vi "Command_verification.vi"(0 "connection ID":refnum<k5>, 1 "System \nSelection":enum32{"Common", "Frosk", "Griffin", "K2"}(ring), 3 "Mode":string(combo)="DProbe", 5 "VTxIndex_In":i8, 6 "probeNumElevAper":i32=1, 9 "time out":i32=40000, 11 "elevAperIndex":i8, 12 "TxpgWaveformStyle":i8) -> (4 "Get_mea_condition":T1 {"RoiLateralSpan" format="%.2f"; "RoiLateralMin" format="%.2f"}, 8 "ElevAperSwitchDepth":sgl, 10 "Result_RLE":bool, 14 "RLE data":string, 15 "Control_elevAperSwitch":bool)   [LabVIEW 2016]
panel:
  out "Dmode(Hout_Lout_Reg)":string[](array[string])
  out "error out 2":errorcluster
  in  "mea_condition_setting":T1 {"RoiLateralMin" format="%.2f"; "RoiLateralSpan" format="%.2f"; "pulseVoltage" format="%.2f"}
  in  "error out":errorcluster
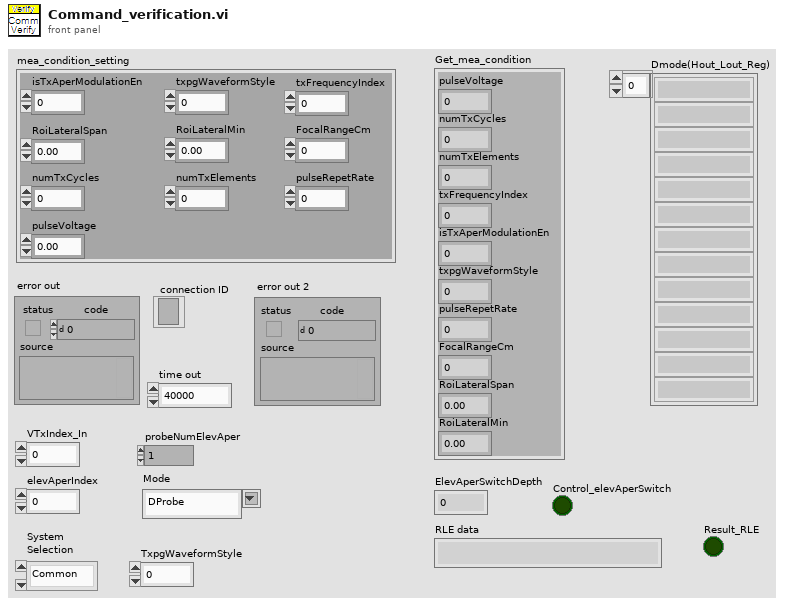
[diagram p1: front panel]
types:
  T1 = cluster{"pulseVoltage":dbl, "numTxCycles":dbl, "numTxElements":i16, "txFrequencyIndex":i32, "isTxAperModulationEn":i16, "txpgWaveformStyle":i16, "pulseRepetRate":dbl, "FocalRangeCm":dbl, "RoiLateralSpan":dbl, "RoiLateralMin":dbl}
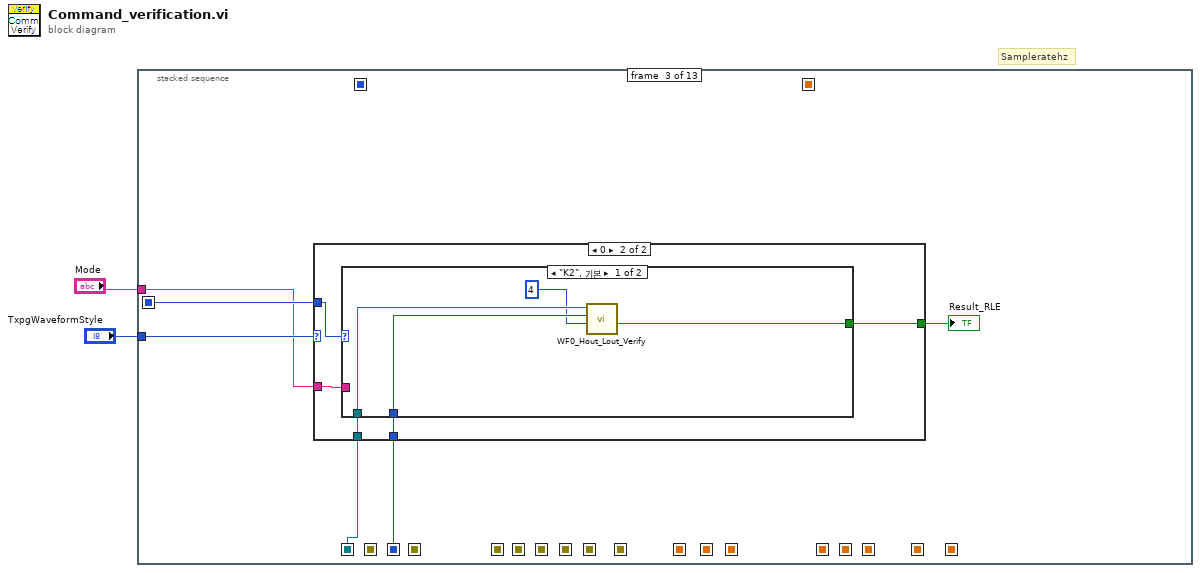
[diagram p0: block diagram]
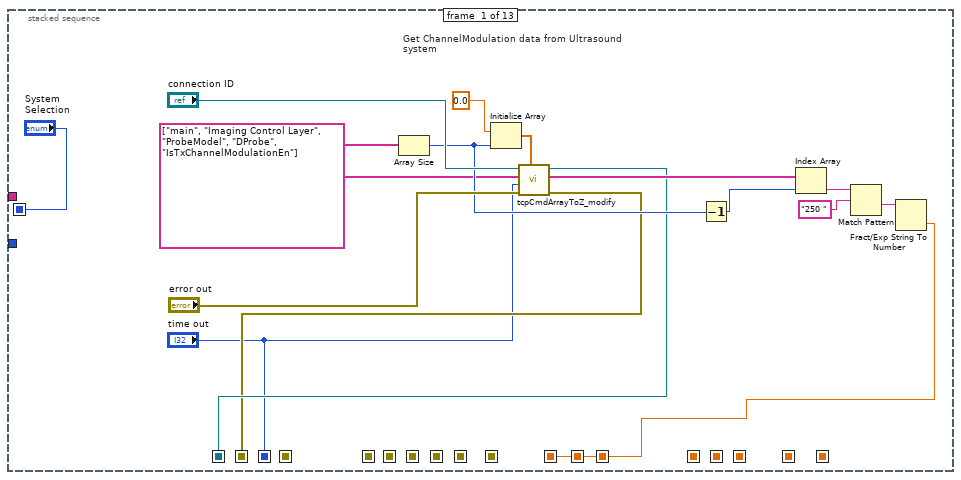
[diagram p2: hidden frame]
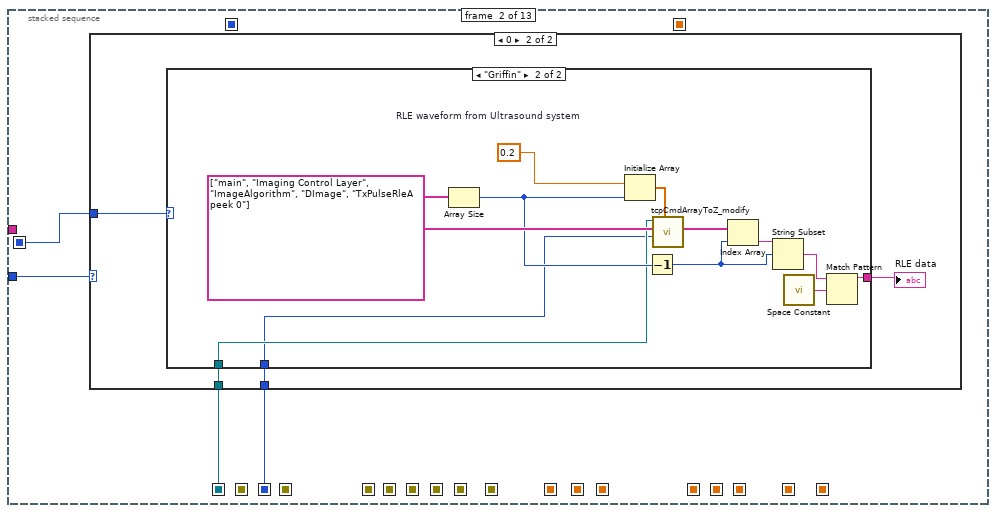
[diagram p3: hidden frame]
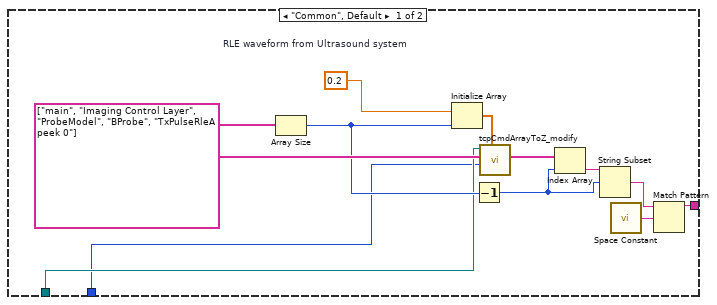
[diagram p5: hidden frame]
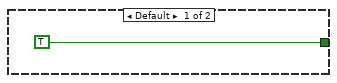
[diagram p6: hidden frame]
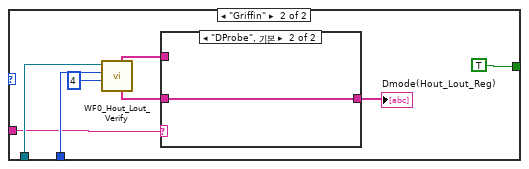
[diagram p7: hidden frame]
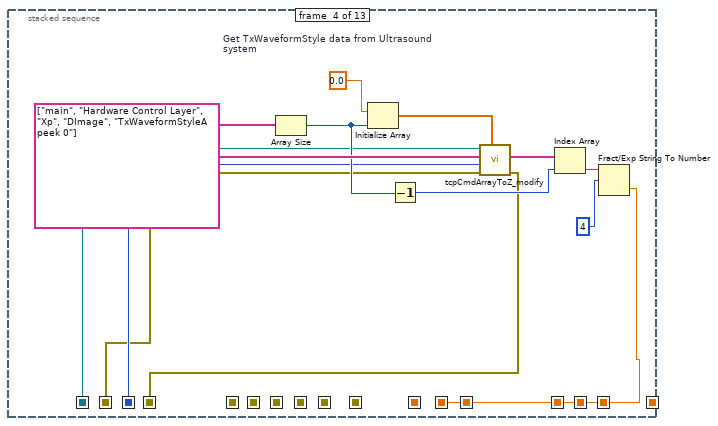
[diagram p9: hidden frame]
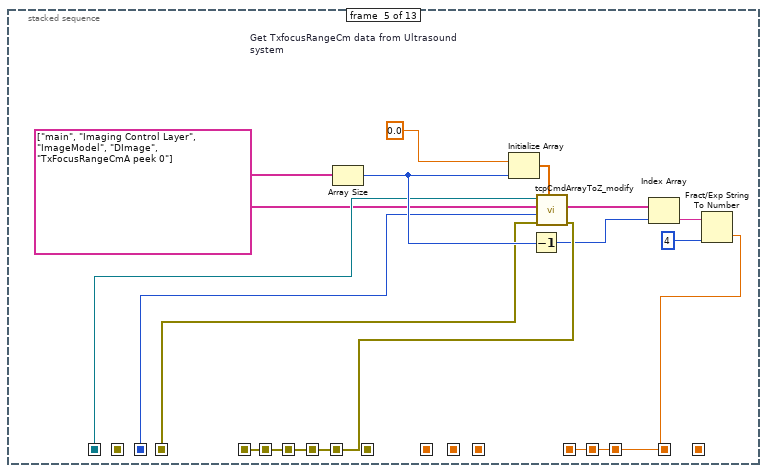
[diagram p10: hidden frame]
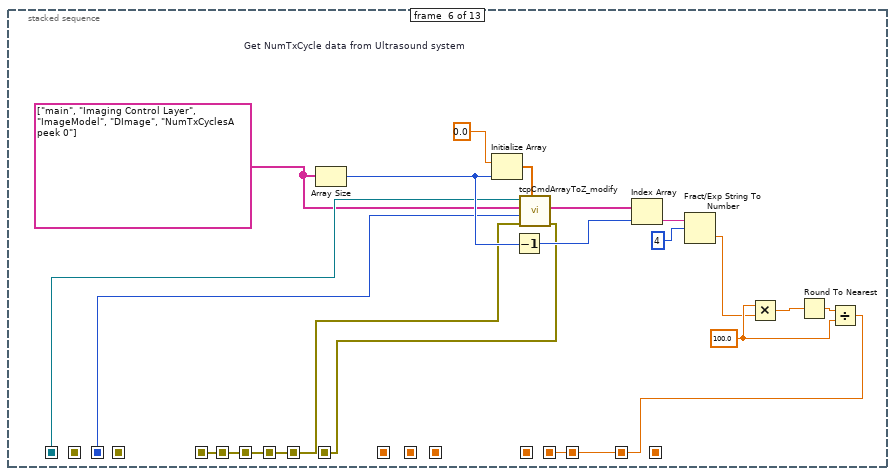
[diagram p11: hidden frame]
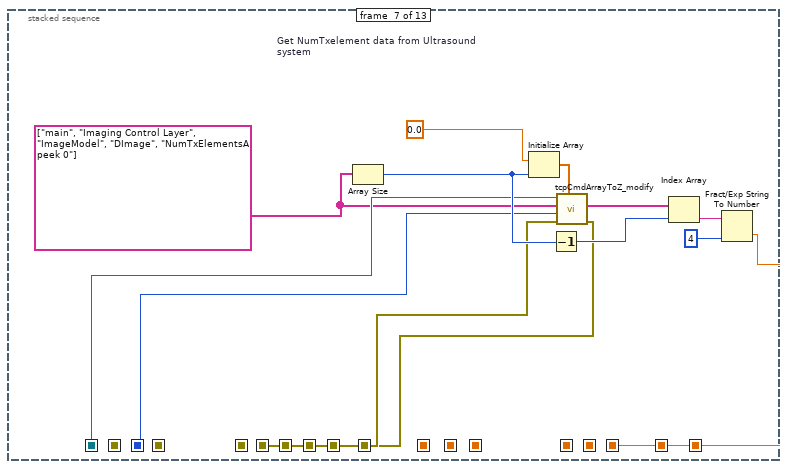
[diagram p12: hidden frame]
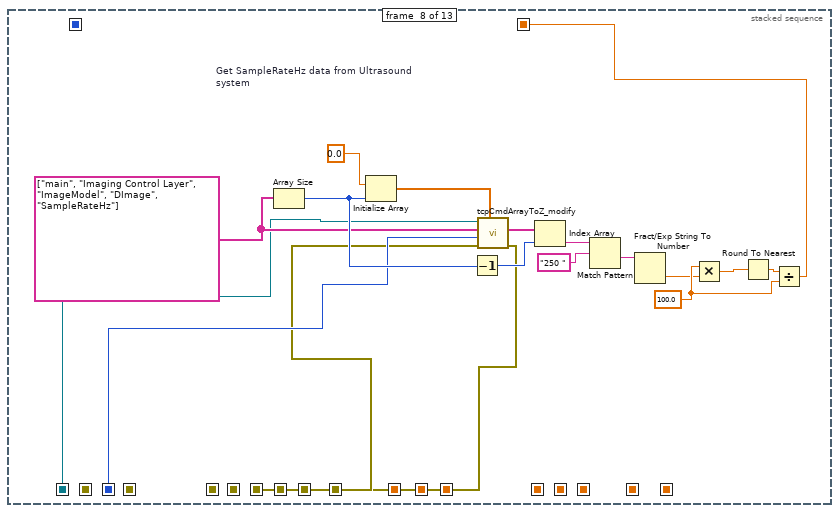
[diagram p13: hidden frame]
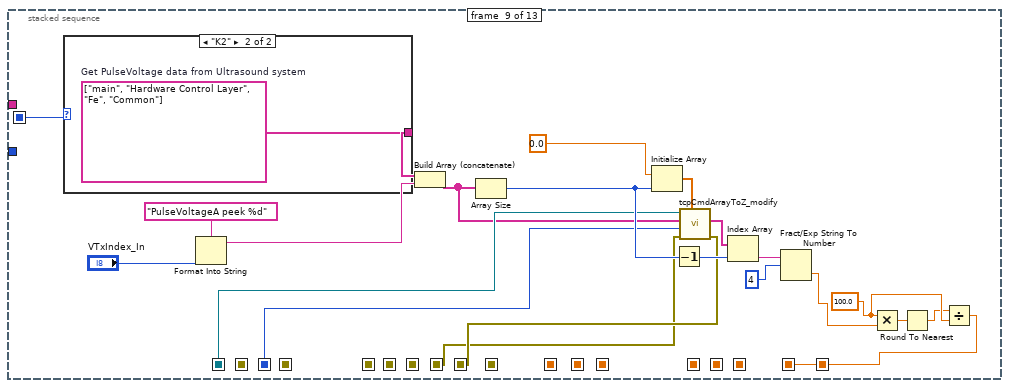
[diagram p14: hidden frame]
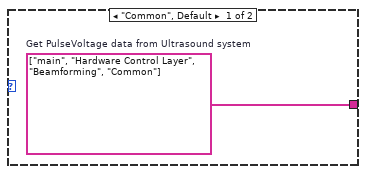
[diagram p15: hidden frame]
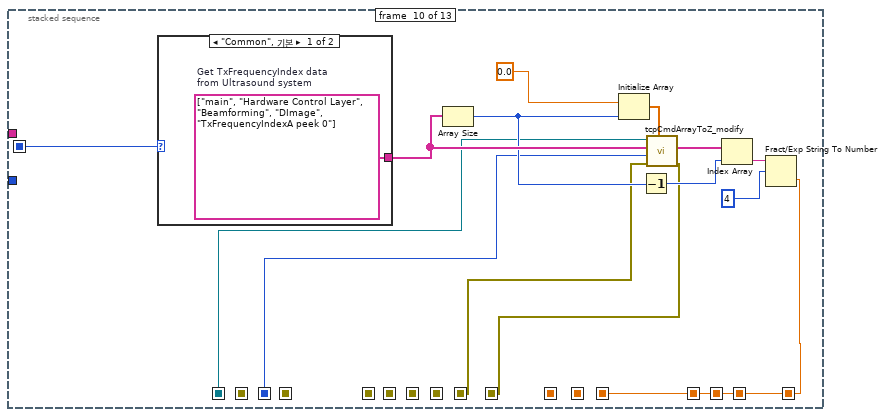
[diagram p16: hidden frame]
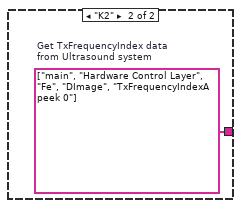
[diagram p17: hidden frame]
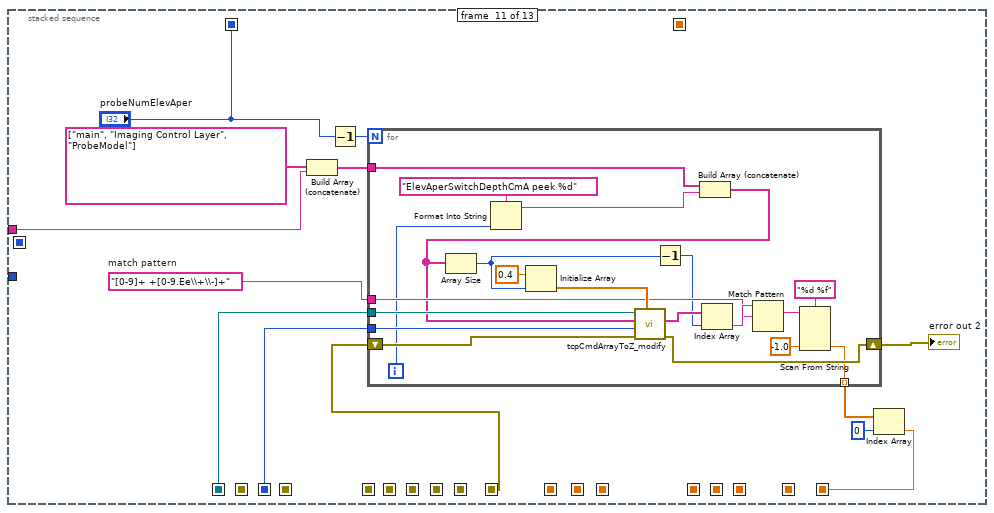
[diagram p18: hidden frame]
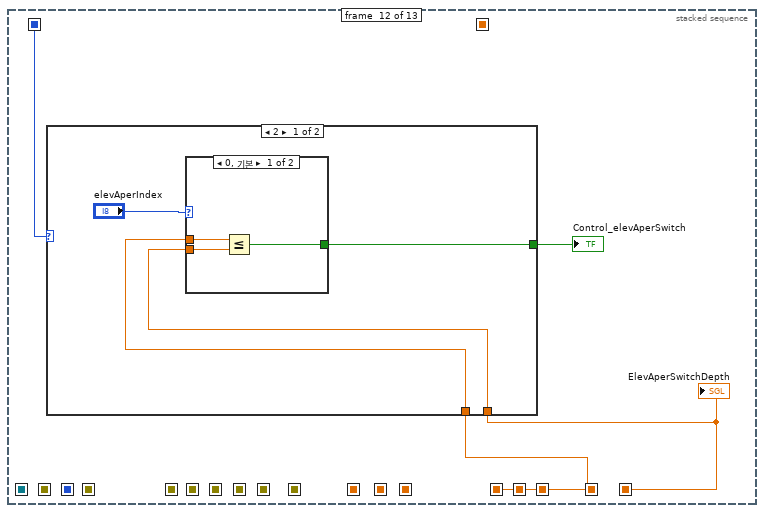
[diagram p19: hidden frame]
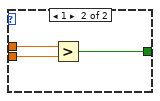
[diagram p20: hidden frame]
diagram:
  # "Sampleratehz"
  n1 = stacked-sequence {
    seq-local: [w11 _ _ _ _ _ _ _ _ _ _ _ _] -> [_ _ _ _ _ _ _ _ _ _ _ _ w247]
    seq-local: [w10 _ _ _ _ _ _ _ _ _ _ _ _] -> [_ w22 w56 w84 w98 w113 w126 w141 w166 w180 w198 _ _]
    seq-local: [w9 _ _ _ _ _ _ _ _ _ _ _ _] -> [_ _ _ w82 _ _ _ _ _ _ _ _ _]
    seq-local: ["time out" _ _ _ _ _ _ _ _ _ _ _ _] -> [_ w21 w55 w83 w97 w112 w125 w140 w165 w179 w197 _ _]
    seq-local: [_ _ _ w79 _ _ _ _ _ _ _ _ _] -> [_ _ _ _ _ _ _ _ _ _ _ _ w246]
    seq-local: [_ _ _ w78 _ _ _ _ _ _ _ _ _] -> [_ _ _ _ w90 _ _ _ _ _ _ _ _]
    seq-local: [_ _ _ _ _ _ _ _ _ w181 _ _ _] -> [_ _ _ _ _ _ _ _ _ _ _ _ w245]
    seq-local: [_ _ _ _ w96 _ _ _ _ _ _ _ _] -> [_ _ _ _ _ w111 _ _ _ _ _ _ _]
    seq-local: [_ _ _ _ w93 _ _ _ _ _ _ _ _] -> [_ _ _ _ _ _ _ _ _ _ _ w226 w244]
    seq-local: [_ _ _ _ _ w110 _ _ _ _ _ _ _] -> [_ _ _ _ _ _ w124 _ _ _ _ _ _]
    seq-local: [_ _ _ _ _ w103 _ _ _ _ _ _ _] -> [_ _ _ _ _ _ _ _ _ _ _ _ w243]
    seq-local: [_ _ _ _ _ _ w123 _ _ _ _ _ _] -> [_ _ _ _ _ _ _ w139 _ _ _ _ _]
    seq-local: [_ _ _ _ _ _ w122 _ _ _ _ _ _] -> [_ _ _ _ _ _ _ _ _ _ _ _ w242]
    seq-local: [_ _ _ _ _ _ _ _ w164 _ _ _ _] -> [_ _ _ _ _ _ _ _ _ w177 _ _ _]
    seq-local: [_ _ _ _ _ _ _ _ w158 _ _ _ _] -> [_ _ _ _ _ _ _ _ _ _ _ _ w241]
    seq-local: [_ _ _ _ _ _ _ w138 _ _ _ _ _] -> [_ _ _ _ _ _ _ _ w157 _ _ _ _]
    seq-local: [_ _ _ _ _ _ _ w133 _ _ _ _ _] -> [_ _ _ _ _ _ _ _ _ _ _ _ w239]
    seq-local: [_ _ _ _ _ _ _ _ _ w176 _ _ _] -> [_ _ _ _ _ _ _ _ _ _ w199 _ _]
    seq-local: [_ _ _ _ _ _ _ _ _ _ w192 _ _] -> [_ _ _ _ _ _ _ _ _ _ _ w225 _]
    seq-local: [_ _ _ _ _ _ _ _ _ _ "probeNumElevAper" _ _] -> [_ _ _ _ _ _ _ _ _ _ _ w227 _]
    seq-local: ["System \nSelection" _ _ _ _ _ _ _ _ _ _ _ _] -> [_ w19 w52 _ _ _ _ _ w151 w175 _ _ _]
    tunnel: "TxpgWaveformStyle" -> [_ w20 w53 _ _ _ _ _ _ _ _ _ _]
    tunnel: "Mode" -> [_ _ w51 _ _ _ _ _ _ _ w191 _ _]
    frame #0 {
      w7 = string[] ["main", "Imaging Control Layer", "ProbeModel", "DProbe", "IsTxChannelModulationEn"]  # Get ChannelModulation data from Ultrasound system
      n2 = Array Size(array=w7) -> (size(s)=w13:i32)
      n3 = Initialize Array(0.0 ("원소"), w13) -> (w15:dbl[])
      n4 = call "tcpCmdArrayToZ_modify.vi"("Delay (sec)"=w15, "error in (no error)"="error out", "Timeout (ms)"="time out", "Command array"=w7, "connection ID in"="connection ID") -> ("error out"=w9:errorcluster, "Receive array"=w14:string[], "connection ID out"=w10:refnum<k5>)  [unwired: 2 in, 2 out]
      n5 = Decrement(x=w13) -> (x-1=w6:i32)
      n6 = Index Array(array=w14, index=w6) -> (element=w12:string)
      n7 = Match Pattern(string=w12, regular expression="250 " ("정규식")) -> (after substring=w5:string)  [unwired: 1 in, 3 out]
      n8 = Fract/Exp String To Number(string=w5) -> (number=w11:dbl)  [unwired: 3 in, 1 out]
    }
    frame #1 {
      n9 = case shown="0" w20 {
        tunnel: w22 -> [_ w26]
        tunnel: w21 -> [_ w25]
        tunnel: w19 -> [_ w23]
        frame Default {
        }
        frame 0 {
          n10 = case shown="\"Griffin\"" w23 {
            tunnel: w26 -> [w31 w43]
            tunnel: w25 -> [w30 w42]
            tunnel: [w27 w39] -> w24
            frame "Common", Default {
              w38 = string[] ["main", "Imaging Control Layer", "ProbeModel", "BProbe", "TxPulseRleA peek 0"]  # RLE waveform from Ultrasound system
              n11 = Array Size(array=w38) -> (size(s)=w34:i32)
              n12 = Initialize Array(0.2 ("원소"), w34) -> (w36:dbl[])
              n13 = Decrement(x=w34) -> (x-1=w32:i32)
              n14 = call "tcpCmdArrayToZ_modify.vi"("Delay (sec)"=w36, "Timeout (ms)"=w30, "Command array"=w38, "connection ID in"=w31) -> ("Receive array"=w35:string[])  [unwired: 3 in, 4 out]
              n15 = Index Array(array=w35, index=w32) -> (element=w33:string)
              n16 = String Subset(string=w33, offset (0)=w32) -> (substring=w29:string)  [unwired: 1 in]
              n17 = call <vilib>:"Space Constant.vi"() -> ("String"=w28:string)
              n18 = Match Pattern(string=w29, regular expression=w28) -> (before substring=w27:string)  [unwired: 1 in, 3 out]
            }
            frame "Griffin" {
              w50 = string[] ["main", "Imaging Control Layer", "ImageAlgorithm", "DImage", "TxPulseRleA peek 0"]  # RLE waveform from Ultrasound system
              n19 = Array Size(array=w50) -> (size(s)=w46:i32)
              n20 = Initialize Array(0.2 ("원소"), w46) -> (w48:dbl[])
              n21 = Decrement(x=w46) -> (x-1=w44:i32)
              n22 = call "tcpCmdArrayToZ_modify.vi"("Delay (sec)"=w48, "Timeout (ms)"=w42, "Command array"=w50, "connection ID in"=w43) -> ("Receive array"=w47:string[])  [unwired: 3 in, 4 out]
              n23 = Index Array(array=w47, index=w44) -> (element=w45:string)
              n24 = String Subset(string=w45, offset (0)=w44) -> (substring=w41:string)  [unwired: 1 in]
              n25 = call <vilib>:"Space Constant.vi"() -> ("String"=w40:string)
              n26 = Match Pattern(string=w41, regular expression=w40) -> (before substring=w39:string)  [unwired: 1 in, 3 out]
            }
          }
          "RLE data" <- w24
        }
      }
    }
    frame #2 {
      n27 = case shown="0" w53 {
        tunnel: w56 -> [_ w62]
        tunnel: w55 -> [_ w61]
        tunnel: [TRUE ("Result_RLE") w60] -> w54
        tunnel: w52 -> [_ w59]
        tunnel: w51 -> [_ w58]
        frame Default {
        }
        frame 0 {
          n28 = case shown="\"K2\", 기본" w59 {
            tunnel: w62 -> [w66 w74]
            tunnel: w61 -> [w65 w73]
            tunnel: [w63 TRUE ("Result_RLE")] -> w60
            tunnel: w58 -> [_ w70]
            frame "K2", Default {
              n29 = call "WF0_Hout_Lout_Verify.vi"("connection ID"=w66, "time out"=w65, "Num_Verify"=4) -> ("Result_RLE"=w63:bool)  [unwired: 1 in, 5 out]
            }
            frame "Griffin" {
              n30 = call "WF0_Hout_Lout_Verify.vi"("connection ID"=w74, "time out"=w73, "Num_Verify"=4) -> ("B-mode(Hout_Lout_Reg)"=w69:string[], "D-mode(Hout_Lout_Reg)"=w68:string[])  [unwired: 1 in, 4 out]
              n31 = case shown="\"DProbe\", 기본" w70 {
                tunnel: w69 -> [w75 _]
                tunnel: w68 -> [_ w76]
                tunnel: [w75 w76] -> w67
                frame "BProbe" {
                }
                frame "DProbe", Default {
                }
              }
              "Dmode(Hout_Lout_Reg)" <- w67
            }
          }
        }
      }
      "Result_RLE" <- w54
    }
    frame #3 {
      w89 = string[] ["main", "Hardware Control Layer", "Xp", "DImage", "TxWaveformStyleA peek 0"]  # Get TxWaveformStyle data from Ultrasound system
      n32 = Array Size(array=w89) -> (size(s)=w85:i32)
      n33 = Initialize Array(0.0 ("원소"), w85) -> (w87:dbl[])
      n34 = Decrement(x=w85) -> (x-1=w80:i32)
      n35 = call "tcpCmdArrayToZ_modify.vi"("Delay (sec)"=w87, "error in (no error)"=w82, "Timeout (ms)"=w83, "Command array"=w89, "connection ID in"=w84) -> ("error out"=w78:errorcluster, "Receive array"=w86:string[])  [unwired: 2 in, 3 out]
      n36 = Index Array(array=w86, index=w80) -> (element=w81:string)
      n37 = Fract/Exp String To Number(string=w81, offset=4 ("오프셋")) -> (number=w79:dbl)  [unwired: 2 in, 1 out]
    }
    frame #4 {
      w92 = string[] ["main", "Imaging Control Layer", "ImageModel", "DImage", "TxFocusRangeCmA peek 0"]  # Get TxfocusRangeCm data from Ultrasound system
      n38 = Array Size(array=w92) -> (size(s)=w100:i32)
      n39 = Initialize Array(0.0 ("원소"), w100) -> (w101:dbl[])
      n40 = Decrement(x=w100) -> (x-1=w94:i32)
      n41 = call "tcpCmdArrayToZ_modify.vi"("Delay (sec)"=w101, "error in (no error)"=w90, "Timeout (ms)"=w97, "Command array"=w92, "connection ID in"=w98) -> ("error out"=w96:errorcluster, "Receive array"=w99:string[])  [unwired: 2 in, 3 out]
      n42 = Index Array(array=w99, index=w94) -> (element=w95:string)
      n43 = Fract/Exp String To Number(string=w95, offset=4 ("오프셋")) -> (number=w93:dbl)  [unwired: 2 in, 1 out]
    }
    frame #5 {
      w106 = 100.0
      w109 = string[] ["main", "Imaging Control Layer", "ImageModel", "DImage", "NumTxCyclesA peek 0"]  # Get NumTxCycle data from Ultrasound system
      n44 = Array Size(array=w109) -> (size(s)=w117:i32)
      n45 = Initialize Array(0.0 ("원소"), w117) -> (w118:dbl[])
      n46 = Decrement(x=w117) -> (x-1=w114:i32)
      n47 = call "tcpCmdArrayToZ_modify.vi"("Delay (sec)"=w118, "error in (no error)"=w111, "Timeout (ms)"=w112, "Command array"=w109, "connection ID in"=w113) -> ("error out"=w110:errorcluster, "Receive array"=w116:string[])  [unwired: 2 in, 3 out]
      n48 = Index Array(array=w116, index=w114) -> (element=w115:string)
      n49 = Fract/Exp String To Number(string=w115, offset=4 ("오프셋")) -> (number=w104:dbl)  [unwired: 2 in, 1 out]
      n50 = Multiply(x=w106, y=w104) -> (x*y=w107:dbl)
      n51 = Round To Nearest(number=w107) -> (nearest integer value=w105:dbl)
      n52 = Divide(x=w105, y=w106) -> (x/y=w103:dbl)
    }
    frame #6 {
      w121 = string[] ["main", "Imaging Control Layer", "ImageModel", "DImage", "NumTxElementsA peek 0"]  # Get NumTxelement data from Ultrasound system
      n53 = Array Size(array=w121) -> (size(s)=w130:i32)
      n54 = Initialize Array(0.0 ("원소"), w130) -> (w131:dbl[])
      n55 = Decrement(x=w130) -> (x-1=w127:i32)
      n56 = call "tcpCmdArrayToZ_modify.vi"("Delay (sec)"=w131, "error in (no error)"=w124, "Timeout (ms)"=w125, "Command array"=w121, "connection ID in"=w126) -> ("error out"=w123:errorcluster, "Receive array"=w129:string[])  [unwired: 2 in, 3 out]
      n57 = Index Array(array=w129, index=w127) -> (element=w128:string)
      n58 = Fract/Exp String To Number(string=w128, offset=4 ("오프셋")) -> (number=w122:dbl)  [unwired: 2 in, 1 out]
    }
    frame #7 {
      w136 = 100.0
      w145 = string[] ["main", "Imaging Control Layer", "ImageModel", "DImage", "SampleRateHz"]  # Get SampleRateHz data from Ultrasound system
      n59 = Array Size(array=w145) -> (size(s)=w147:i32)
      n60 = Initialize Array(0.0 ("원소"), w147) -> (w149:dbl[])
      n61 = Decrement(x=w147) -> (x-1=w144:i32)
      n62 = call "tcpCmdArrayToZ_modify.vi"("Delay (sec)"=w149, "error in (no error)"=w139, "Timeout (ms)"=w140, "Command array"=w145, "connection ID in"=w141) -> ("error out"=w138:errorcluster, "Receive array"=w148:string[])  [unwired: 2 in, 3 out]
      n63 = Index Array(array=w148, index=w144) -> (element=w146:string)
      n64 = Match Pattern(string=w146, regular expression="250 " ("정규식")) -> (after substring=w143:string)  [unwired: 1 in, 3 out]
      n65 = Fract/Exp String To Number(string=w143) -> (number=w134:dbl)  [unwired: 3 in, 1 out]
      n66 = Multiply(x=w136, y=w134) -> (x*y=w137:dbl)
      n67 = Round To Nearest(number=w137) -> (nearest integer value=w135:dbl)
      n68 = Divide(x=w135, y=w136) -> (x/y=w133:dbl)
    }
    frame #8 {
      w161 = 100.0
      n69 = case shown="\"K2\"" w151 {
        tunnel: [w173 w174] -> w155
        frame "Common", Default {
          w173 = string[] ["main", "Hardware Control Layer", "Beamforming", "Common"]  # Get PulseVoltage data from Ultrasound system
        }
        frame "K2" {
          w174 = string[] ["main", "Hardware Control Layer", "Fe", "Common"]  # Get PulseVoltage data from Ultrasound system
        }
      }
      n70 = Format Into String(format string="PulseVoltageA peek %d" ("Format String"), "VTxIndex_In") -> (resulting string=w154:string)  [unwired: 2 in, 1 out]
      n71 = Build Array (concatenate)(w155, w154) -> (w153:string[])
      n72 = Array Size(array=w153) -> (size(s)=w170:i32)
      n73 = Initialize Array(0.0 ("원소"), w170) -> (w171:dbl[])
      n74 = Decrement(x=w170) -> (x-1=w167:i32)
      n75 = call "tcpCmdArrayToZ_modify.vi"("Delay (sec)"=w171, "error in (no error)"=w157, "Timeout (ms)"=w165, "Command array"=w153, "connection ID in"=w166) -> ("error out"=w164:errorcluster, "Receive array"=w169:string[])  [unwired: 2 in, 3 out]
      n76 = Index Array(array=w169, index=w167) -> (element=w168:string)
      n77 = Fract/Exp String To Number(string=w168, offset=4 ("오프셋")) -> (number=w159:dbl)  [unwired: 2 in, 1 out]
      n78 = Multiply(x=w161, y=w159) -> (x*y=w162:dbl)
      n79 = Round To Nearest(number=w162) -> (nearest integer value=w160:dbl)
      n80 = Divide(x=w160, y=w161) -> (x/y=w158:dbl)
    }
    frame #9 {
      n81 = case shown="\"Common\", 기본" w175 {
        tunnel: [w189 w190] -> w188
        frame "Common", Default {
          w189 = string[] ["main", "Hardware Control Layer", "Beamforming", "DImage", "TxFrequencyIndexA peek 0"]  # Get TxFrequencyIndex data from Ultrasound system
        }
        frame "K2" {
          w190 = string[] ["main", "Hardware Control Layer", "Fe", "DImage", "TxFrequencyIndexA peek 0"]  # Get TxFrequencyIndex data from Ultrasound system
        }
      }
      n82 = Array Size(array=w188) -> (size(s)=w184:i32)
      n83 = Initialize Array(0.0 ("원소"), w184) -> (w186:dbl[])
      n84 = Decrement(x=w184) -> (x-1=w182:i32)
      n85 = call "tcpCmdArrayToZ_modify.vi"("Delay (sec)"=w186, "error in (no error)"=w177, "Timeout (ms)"=w179, "Command array"=w188, "connection ID in"=w180) -> ("error out"=w176:errorcluster, "Receive array"=w185:string[])  [unwired: 2 in, 3 out]
      n86 = Index Array(array=w185, index=w182) -> (element=w183:string)
      n87 = Fract/Exp String To Number(string=w183, offset=4 ("오프셋")) -> (number=w181:dbl)  [unwired: 2 in, 1 out]
    }
    frame #10 {
      w200 = "[0-9]+ +[0-9.Ee\\+\\-]+"  # match pattern
      n88 = Build Array (concatenate)(string[] ["main", "Imaging Control Layer", "ProbeModel"] ("menu cmds for NumElevAper\nmain Imaging Control Layer ProbeRootPc CommonProbe"), w191) -> (w201:string[])
      n89 = Decrement(x="probeNumElevAper") -> (x-1=w203:i32)
      n90 = for {
        N: w203 -> [_]
        tunnel: w198 -> [w222]
        tunnel: w197 -> [w221]
        shift-right: [w216] -> w196
        shift-left: w199 -> [w220]
        tunnel: w200 -> [w214]
        tunnel: [w205] -> w194 mode=indexing
        tunnel: w201 -> [w210]
        i -> [w211]
        n91 = Format Into String(format string="ElevAperSwitchDepthCmA peek %d" ("Format String"), w211) -> (resulting string=w207:string)  [unwired: 2 in, 1 out]
        n92 = Build Array (concatenate)(w210, w207) -> (w209:string[])
        n93 = Array Size(array=w209) -> (size(s)=w213:i32)
        n94 = Initialize Array(0.4, w213) -> (w223:dbl[])
        n95 = call "tcpCmdArrayToZ_modify.vi"("Delay (sec)"=w223, "error in (no error)"=w220, "Timeout (ms)"=w221, "Command array"=w209, "connection ID in"=w222) -> ("error out"=w216:errorcluster, "Receive array"=w215:string[])  [unwired: 2 in, 3 out]
        n96 = Decrement(x=w213) -> (x-1=w212:i32)
        n97 = Index Array(array=w215, index=w212) -> (element=w217:string)
        n98 = Match Pattern(string=w217, regular expression=w214) -> (match substring=w219:string)  [unwired: 1 in, 3 out]
        n99 = Scan From String(format string="%d %f" ("Format String"), input string=w219, default 2=sgl -1.0 ("Default Value 2")) -> (output 2=w205:sgl)  [unwired: 4 in, 3 out]
      }
      "error out 2" <- w196
      n100 = Index Array(array=w194, index=0 ("인덱스")) -> (element=w192:sgl)
    }
    frame #11 {
      n101 = case shown="2" w227 {
        tunnel: w226 -> [w230 _]
        tunnel: w225 -> [w229 _]
        tunnel: [w228 TRUE] -> w224
        frame 2 {
          n102 = case shown="0, 기본" "elevAperIndex" {
            tunnel: w230 -> [w234 w237]
            tunnel: w229 -> [w233 w236]
            tunnel: [w232 w235] -> w228
            frame 0, Default {
              n103 = Less Or Equal?(x=w234, y=w233) -> (x <= y?=w232:bool)
            }
            frame 1 {
              n104 = Greater?(x=w237, y=w236) -> (0:w235:bool)
            }
          }
        }
        frame 1, Default {
        }
      }
      "Control_elevAperSwitch" <- w224
      "ElevAperSwitchDepth" <- w225
    }
    frame #12 {
      n105 = Bundle By Name(cluster="mea_condition_setting", "pulseVoltage"=w241, "numTxCycles"=w243, "numTxElements"=w242, "txFrequencyIndex"=w245, "isTxAperModulationEn"=w247, "txpgWaveformStyle"=w246, "FocalRangeCm"=w244, "pulseRepetRate"=w239) -> (→"Get_mea_condition":T1)
    }
  }
